vi "SPC_read_fifo.vi"(8 "Error In":errorcluster, 9 "Input Count":i32=1002 max=3200064 step=1, 10 "Module No":i16 min=0 max=7 step=1, 11 "DLL Path":path) -> (0 "Error Out":errorcluster, 2 "Module No":i16 min=0 max=7 step=1, 3 "DLL Path":path, 4 "Output Count":u32 step=1, 5 "Data Buffer":u16[](array[numeric]))   [LabVIEW 2023]
doc: "The procedure reads data from the FIFO memory of SPC modules SPC6x0/13x/830/140/15x/160 and has no effect for other SPC module types. Because of hardware differences the procedure action is different for different SPC module types.\nFor SPC600(630) modules:\nBefore calling the function FIFO mode must be set by calling function SPC_set_parameter to change parameter MODE to one of two possible FIFO modes: FIFO_48 (48 bits frame) or FIFO_32 (32 bits frame) (fifo mode values are defined in spcm_def.h file).\nFor FIFO_48 mode the function reads 48-bits frames from the FIFO memory and writes them to the buffer 'data' until the FIFO is empty or 'Count' number of 16-bit words was already written. The 'Count' variable is filled on exit with the number of 16-bit words written to the buffer.\nFor FIFO_32 mode the function reads 32-bits frames from the FIFO memory and writes them to the buffer 'data' until the FIFO is empty or 'Count' number of 16-bit words was already written. The 'Count' variable is filled on exit with the number of 16-bit words written to the buffer. Subsequent frames which don't contain valid data but only macro time overflow information are compressed to one frame which contains the number of macro time overflows in the bits 29:0. It enables a correct macro time calculation and eliminates invalid data frames from the buffer.\nFor SPC13x/830/140/15x/160/930 modules:\nBefore calling the function FIFO mode must be set by calling function SPC_set_parameter to change parameter MODE to FIFO mode (32 bits frame different than for SPC6x0 modules) (fifo mode values are defined in spcm_def.h file). After setting FIFO mode SPC module memory has FIFO structure. SPC_read_fifo function reads 32-bits frames from the FIFO memory and writes them to the buffer 'data' until the FIFO is empty or 'Count' number of 16-bit words was already written. \nThe 'Count' variable is filled on exit with the number of 16-bit words written to the buffer. Subsequent frames which don't contain valid data ( photons or markers ) but only macro time overflow information are compressed to one frame which contains the number of macro time overflows in the bits 29:0. It enables a correct macro time calculation and eliminates invalid data frames from the buffer.\nFor SPC830/140/15x/160 modules in FIFO_32M ( FIFO IMAGE) mode:\nworks as above with a difference after calling SPC_stop_measurement - function will return 1 ( instead of 0 ) when photons are read up to stop pointer in FIFO - see explanation in SPC_stop_measurement function description \nPlease make sure that the buffer 'data' be allocated with enough memory for the expected number of frames (at least 'Count' 16-bit words).\n\n<b>Attention:</b> this VI runs Inline to increase performance of memory allocation\n\ninfo@becker-hickl.com"
panel:
  # "Attention: this VI runs Inline to increase memory allocation performance"
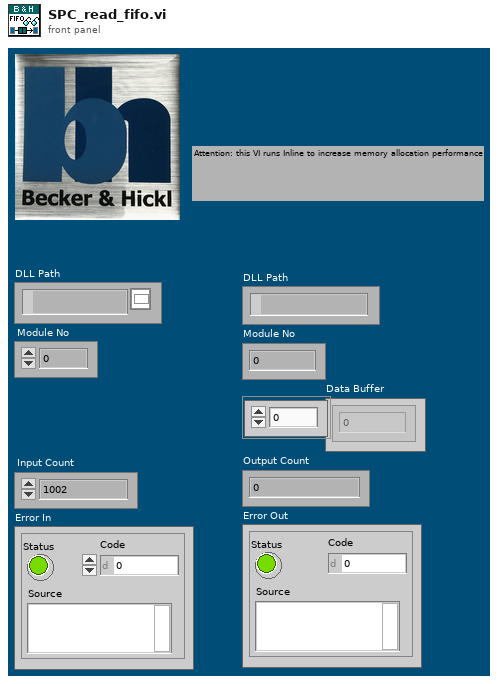
[diagram p1: front panel]
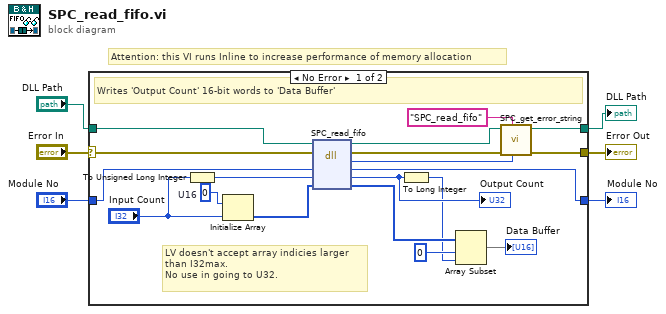
[diagram p0: block diagram]
diagram:
  # "Attention: this VI runs Inline to increase performance of memory allocation"
  n1 = case shown="No Error" "Error In" {
    selector: "Error In" -> [w20 w28]
    tunnel: [w17 w28] -> w6
    tunnel: "DLL Path" -> [w19 w27]
    tunnel: [w14 w27] -> w3
    tunnel: "Module No" -> [w13 w26]
    tunnel: [w12 w26] -> w1
    frame No Error {
      w24 = u16 0  # U16
      # "LV doesn't accept array indicies larger \nthan I32max.\nNo use in going to U32."
      # "Writes 'Output Count' 16-bit words to 'Data Buffer'"
      n2 = To Unsigned Long Integer(number="Input Count") -> (unsigned 32bit integer=w9:u32)
      n3 = Initialize Array "Initialize Array"(w24, "Input Count") -> (w25:u16[])
      n4 = dll-call lib="D:/spcm/lib/lab_view/lv10.0/spcm32.dll" fn="SPC_read_fifo"(path in=w19, error in=w20, "mod_no"=w13, "count"=w9, "data"=w25) -> (path out=w15:path, error out=w18:errorcluster, "return type"=w16:i16, "mod_no"=w12:i16, "count"=w22:u32, "data"=w21:u16[])  [unwired: 1 in]
      "Output Count" <- w22
      n5 = To Long Integer(number=w22) -> (32bit integer=w11:i32)
      n6 = Array Subset(array=w21, index=0, length=w11) -> (→"Data Buffer":u16[])
      n7 = call "SPC_get_error_string.vi"("ErrorID"=w16, "VI-name if Inline"="SPC_read_fifo", "Error In"=w18, "DLL Path"=w15) -> ("Error Out"=w17:errorcluster, "DLL Path"=w14:path)  [unwired: 5 in, 1 out]
    }
    frame Error {
    }
  }
  "Error Out" <- w6
  "DLL Path" <- w3
  "Module No" <- w1
